vi "FeedBack Chanel.vi"(0 "Test Name":string, 5 "Channels (Int)":i32[](array[numeric]), 7 "FeedBack Channel":string[](array[string])=["fgdgfvcbc", "vnfhgjkn", "21354682"], 9 "Wait/Poll (ms)":u32, 11 "Parameter":u8) -> (4 "Out":i32, 6 "Array":bool[](array[boolean]), 8 "Fail":bool, 12 "Input Status":bool[](array[boolean]), 13 "Channel No":i32[](array[numeric]))   [LabVIEW 2015]
uses:
  Galobal variable_TI.vi
  Project Setup/Globle Variable/GR_Servo.vi
panel:
  in  "Load":bool
  out "Pokayoka Result":cluster{"Sensor Name":string, "Boolean":bool}[](array[cluster])
  out "output array":bool[](array[boolean])
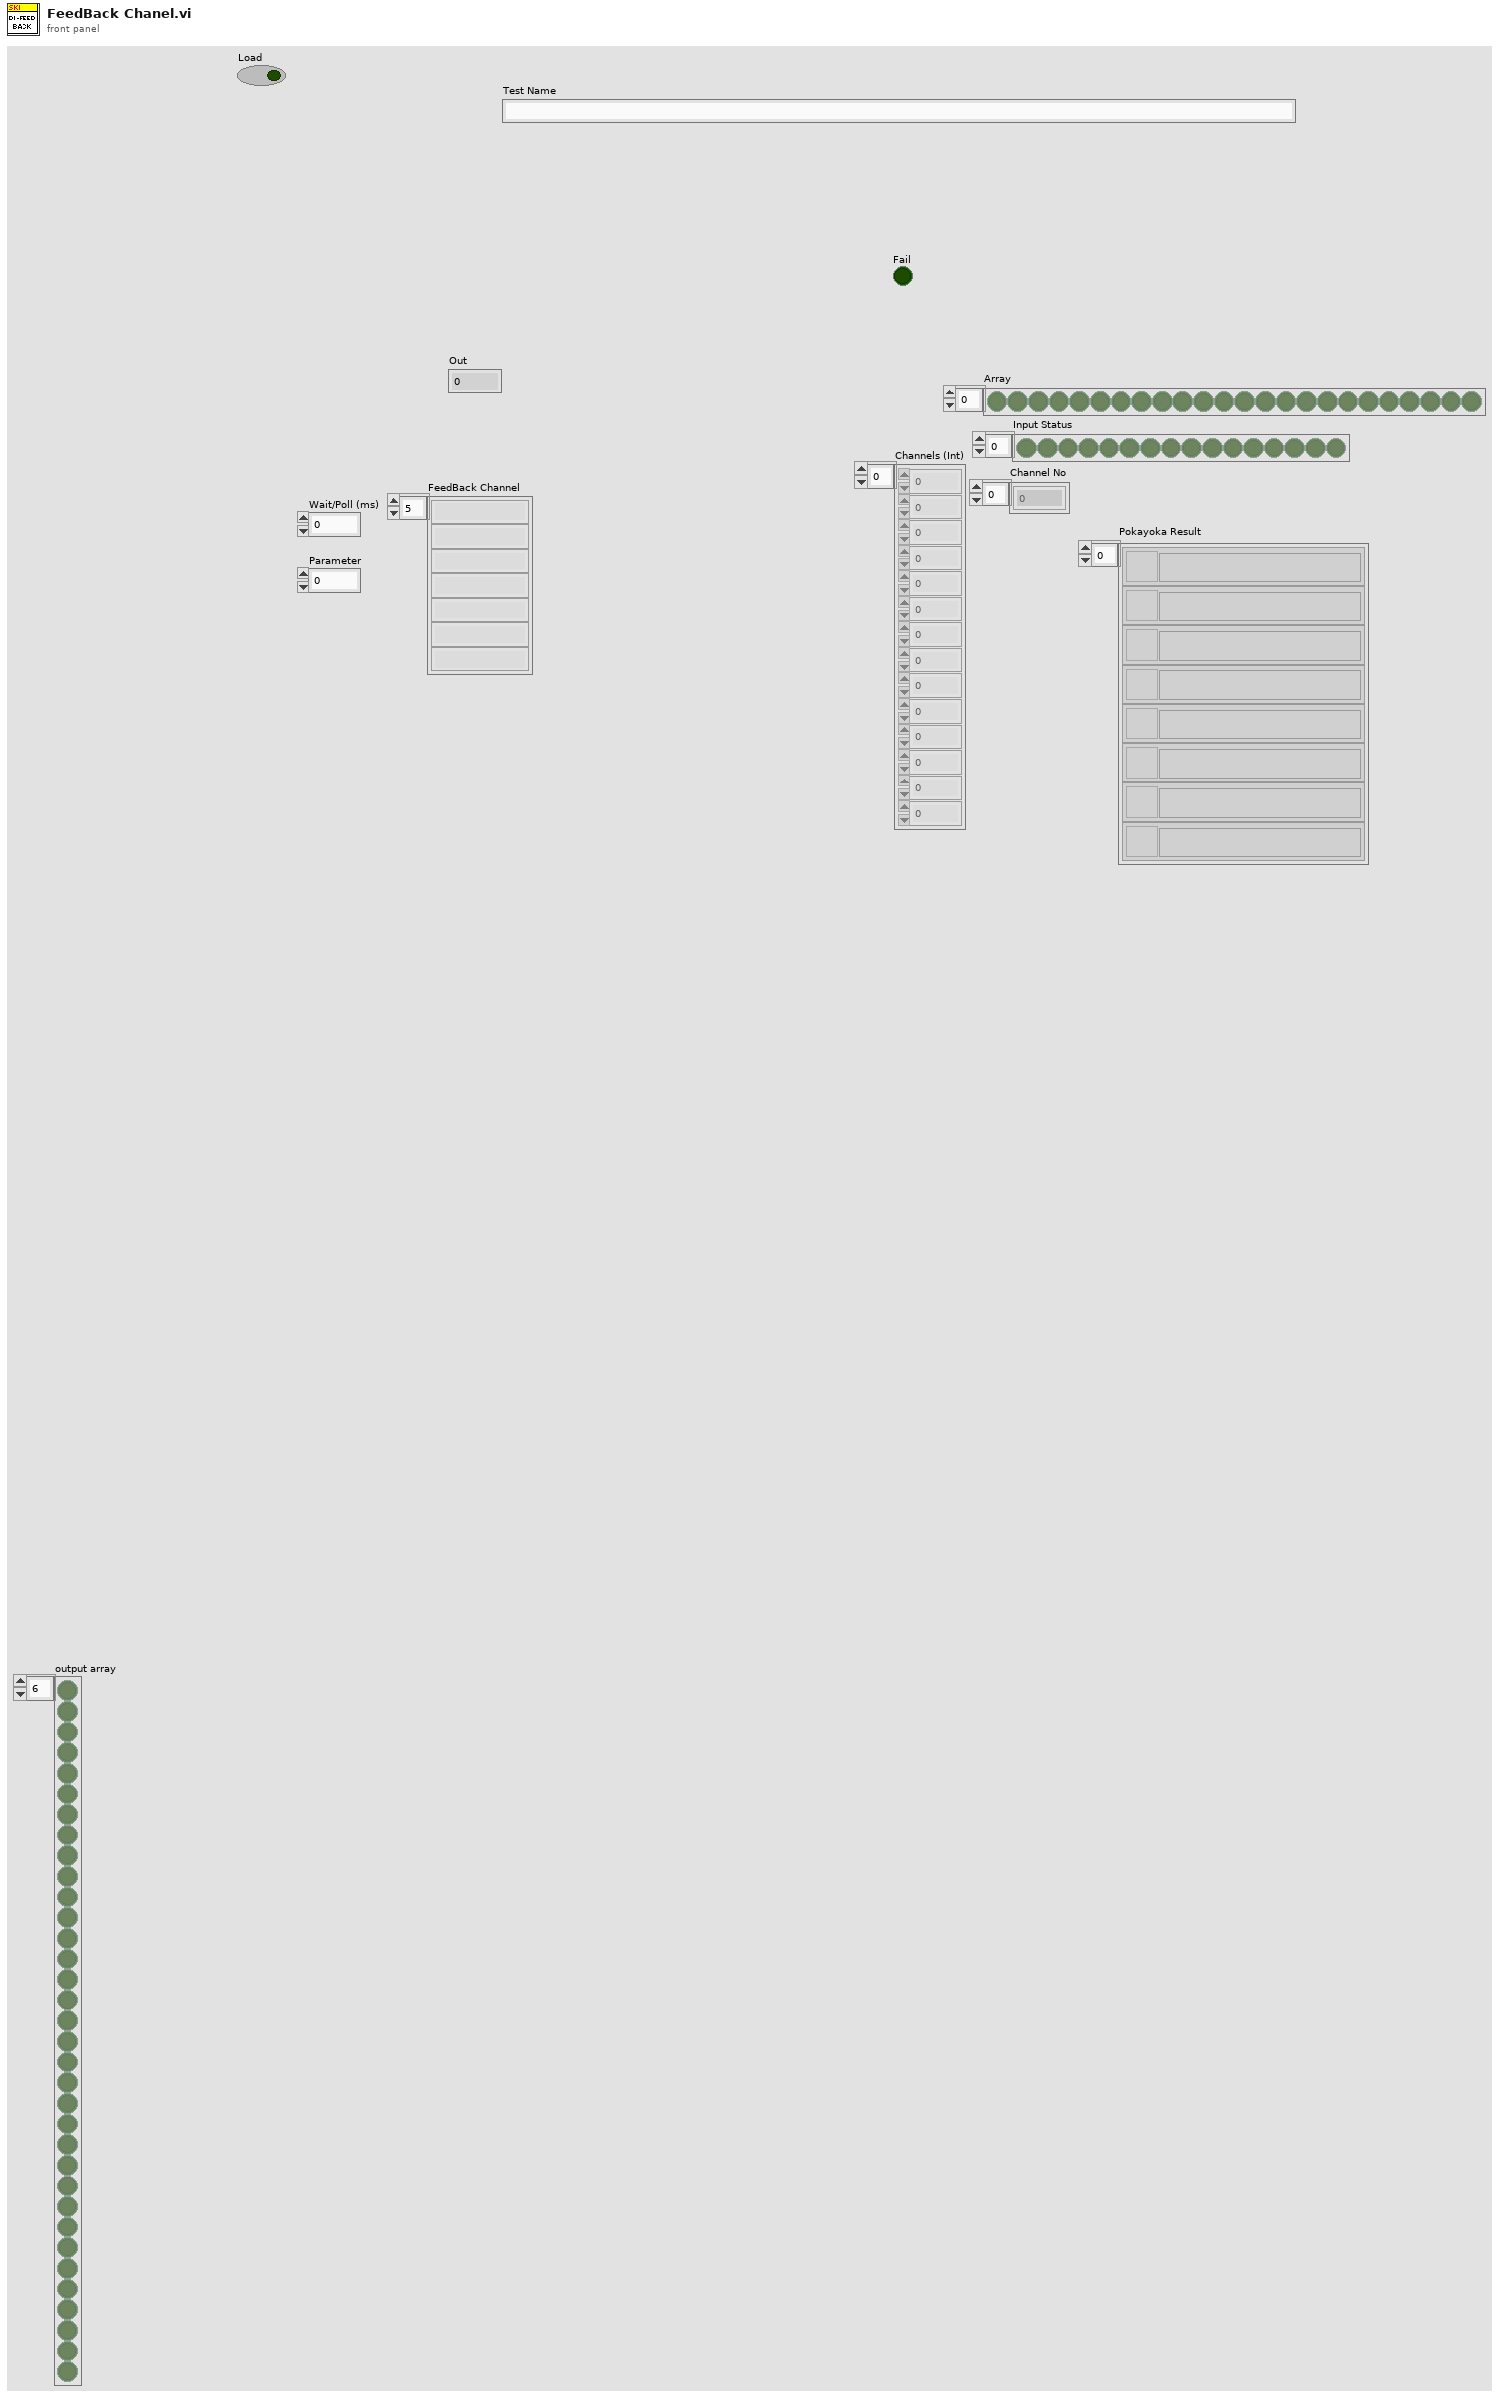
[diagram p1: front panel]
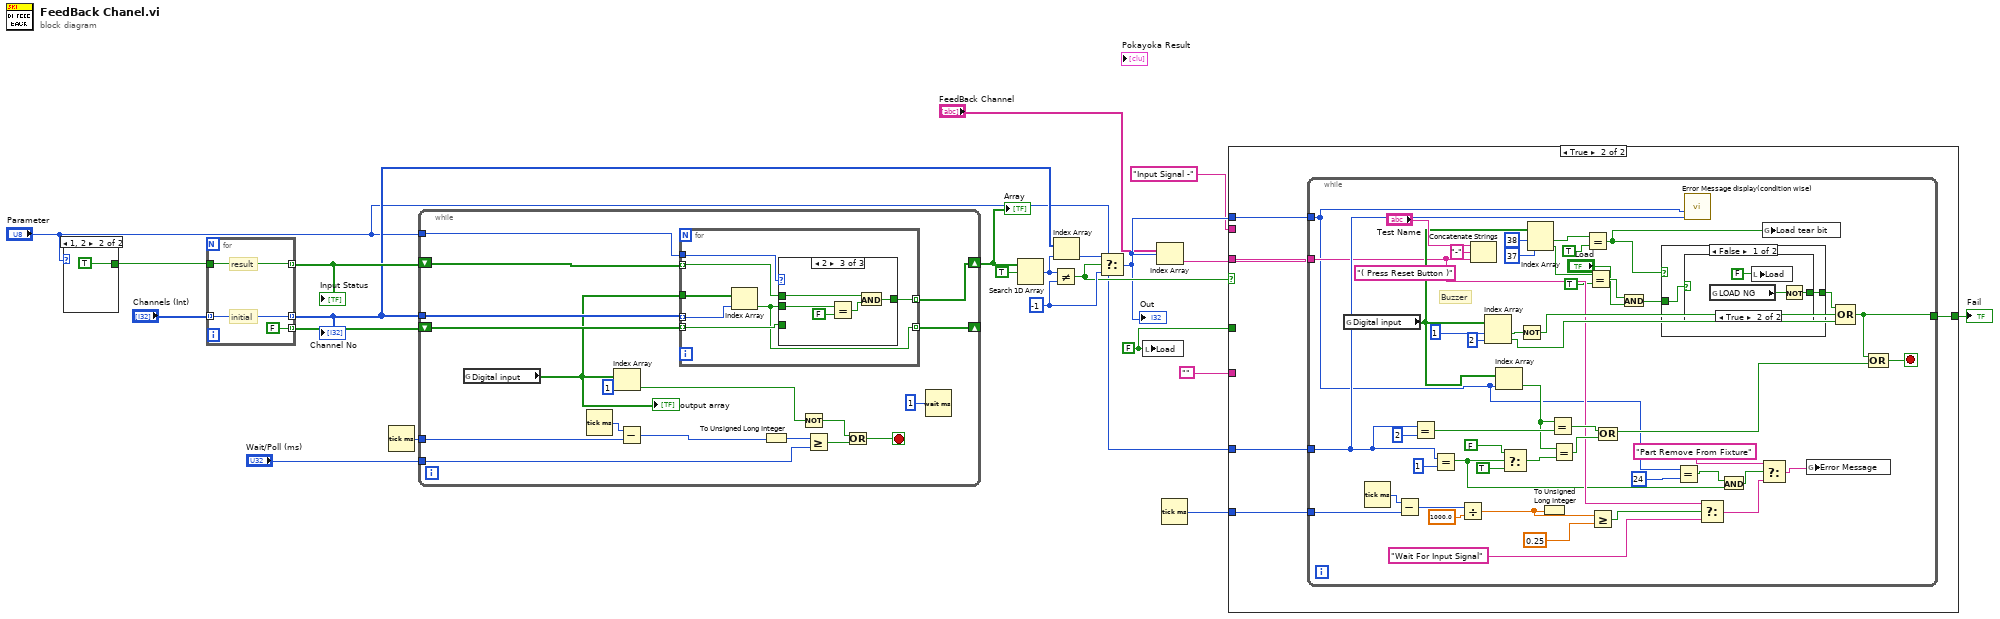
[diagram p0: block diagram]
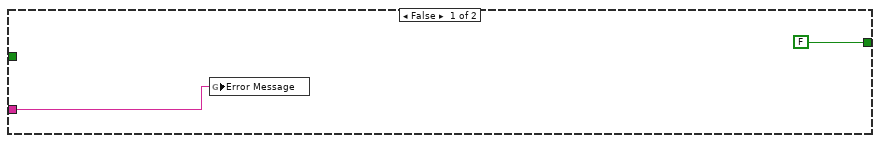
[diagram p2: hidden frame]
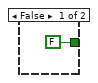
[diagram p3: hidden frame]
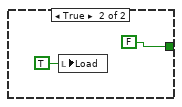
[diagram p4: hidden frame]
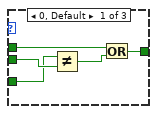
[diagram p5: hidden frame]
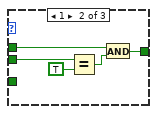
[diagram p6: hidden frame]
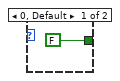
[diagram p7: hidden frame]
diagram:
  w1 = FALSE ("Load")
  w22 = -1 ("y")
  n1 = case shown="1, 2" "Parameter" {
    tunnel: [FALSE TRUE] -> w13
    frame 0, Default {
    }
    frame 1, 2 {
    }
  }
  n2 = for {
    tunnel: [w27] -> w8 mode=indexing
    tunnel: w13 -> [w27]
    tunnel: "Channels (Int)" -> [w26] mode=indexing
    tunnel: [w26] -> w7 mode=indexing
    tunnel: [FALSE] -> w17 mode=indexing
    # "result"
    # "initial"
  }
  "Input Status" <- w8
  "Channel No" <- w7
  n3 = Tick Count (ms)() -> (millisecond timer value=w16:u32)
  n4 = while {
    tunnel: "Wait/Poll (ms)" -> [w33]
    tunnel: w16 -> [w44]
    tunnel: w7 -> [w42]
    tunnel: "Parameter" -> [w41]
    shift-right: [w40] -> w19
    shift-left: w8 -> [w38]
    shift-right: [w39] -> _
    shift-left: w17 -> [w37]
    stop <- w35 stop-if-true
    n5 = global read "Galobal variable_TI.vi" "Digital input"() -> (w29:bool[])
    "output array" <- w29
    n6 = Tick Count (ms)() -> (millisecond timer value=w45:u32)
    n7 = Index Array(array=w29, index=1) -> (element=w31:bool)
    n8 = Subtract(x=w45, y=w44) -> (x-y=w28:u32)
    n9 = for {
      tunnel: w37 -> [w47] mode=indexing
      tunnel: w38 -> [w49] mode=indexing
      tunnel: w29 -> [w52]
      tunnel: w42 -> [w51] mode=indexing
      tunnel: w41 -> [w50]
      tunnel: [w48] -> w40 mode=indexing
      tunnel: [w46] -> w39 mode=indexing
      n10 = Index Array(array=w52, index=w51) -> (element=w46:bool)
      n11 = case shown="2" w50 {
        tunnel: w46 -> [w57 w60 w67]
        tunnel: w49 -> [w55 w59 w64]
        tunnel: [w53 w58 w63] -> w48
        tunnel: w47 -> [w56 _ _]
        frame 0, Default {
          n12 = Not Equal?(x=w56, y=w57) -> (x != y?=w54:bool)
          n13 = Or(x=w55, y=w54) -> (x .or. y?=w53:bool)
        }
        frame 1 {
          n14 = Equal?(x=w60, y=TRUE) -> (x = y?=w61:bool)
          n15 = And(x=w59, y=w61) -> (x .and. y?=w58:bool)
        }
        frame 2 {
          n16 = Equal?(x=w67, y=FALSE) -> (x = y?=w65:bool)
          n17 = And(x=w64, y=w65) -> (x .and. y?=w63:bool)
        }
      }
    }
    n18 = To Unsigned Long Integer(number=w28) -> (unsigned 32bit integer=w43:u32)
    n19 = Not(x=w31) -> (.not. x?=w32:bool)
    n20 = Greater Or Equal?(x=w43, y=w33) -> (x >= y?=w36:bool)
    n21 = Or(x=w32, y=w36) -> (x .or. y?=w35:bool)
    n22 = Wait (ms)(milliseconds to wait=u32 1) -> ()  [unwired: 1 out]
  }
  "Array" <- w19
  n23 = Search 1D Array(1D array=w19, element=TRUE) -> (index of element=w20:i32)  [unwired: 1 in]
  n24 = Not Equal?(x=w20, y=w22) -> (x != y?=w12:bool)
  n25 = Index Array(array=w7, index=w20) -> (element=w21:i32)
  n26 = Select(t=w21, s=w12, f=w22) -> (s? t:f=w11:i32)
  "Out" <- w11
  n27 = local write "Load"(w1) -> ()
  n28 = Index Array(array="FeedBack Channel", index=w11) -> (element=w10:string)
  n29 = Tick Count (ms)() -> (millisecond timer value=w5:u32)
  n30 = case shown="True" w12 {
    tunnel: w11 -> [_ w73]
    tunnel: w10 -> [_ w74]
    tunnel: "Input Signal -" ("string") -> [_ _]
    tunnel: w5 -> [_ w72]
    tunnel: "" -> [w69 _]
    tunnel: [FALSE w71] -> w2
    tunnel: "Parameter" -> [_ w70]
    tunnel: w1 -> [_ _]
    frame False {
      n31 = global write "GR_Servo.vi" "Error Message"(w69) -> ()
    }
    frame True {
      n32 = while {
        tunnel: w74 -> [w92]
        tunnel: w73 -> [w90]
        tunnel: w72 -> [w117]
        tunnel: [w98] -> w71
        tunnel: w70 -> [w97]
        stop <- w122 stop-if-true
        (unwired) "( Press Reset Button )" ("string")
        # "Buzzer"
        n33 = global read "Galobal variable_TI.vi" "Digital input"() -> (w96:bool[])
        n34 = Tick Count (ms)() -> (millisecond timer value=w120:u32)
        n35 = Subtract(x=w120, y=w117) -> (x-y=w119:u32)
        n36 = Equal?(x=w97, y=u8 2) -> (x = y?=w103:bool)
        n37 = Equal?(x=w97, y=u8 1) -> (x = y?=w88:bool)
        n38 = Divide(x=w119, y=1000.0) -> (x/y=w91:dbl)
        n39 = Concatenate Strings("Test Name", "-" ("string"), w92) -> ()  [unwired: 1 out]
        n40 = Index Array(array=w96, index #1=1 ("index"), index #2=2 ("index")) -> (element #1=w112:bool, element #2=w109:bool)
        n41 = Index Array(array=w96, index=w90) -> (element=w102:bool)
        n42 = Select(t=FALSE, s=w88, f=TRUE) -> (s? t:f=w104:bool)
        n43 = Not(x=w112) -> (.not. x?=w110:bool)
        n44 = Index Array(array=w96, index #1=38 ("index"), index #2=37 ("index")) -> (element #1=w94:bool, element #2=w79:bool)
        n45 = To Unsigned Long Integer(number=w91) -> ()  [unwired: 1 out]
        n46 = Equal?(x=w102, y=w103) -> (x = y?=w101:bool)
        n47 = Equal?(x=w102, y=w104) -> (x = y?=w100:bool)
        n48 = Equal?(x=w94, y=TRUE) -> (x = y?=w76:bool)
        n49 = Equal?(x=w79, y=TRUE) -> (x = y?=w78:bool)
        n50 = Greater Or Equal?(x=w91, y=0.25) -> (x >= y?=w115:bool)
        n51 = Compound Arithmetic op=OR(w101, w100) -> (w99:bool)
        n52 = And(x=w78, y="Load") -> (x .and. y?=w75:bool)
        n53 = case shown="False" w76 {
          tunnel: [w125 FALSE ("LOAD NG")] -> w82
          tunnel: w75 -> [w124 _]
          frame False {
            n54 = case shown="True" w124 {
              tunnel: [FALSE w128] -> w125
              frame False {
              }
              frame True {
                n55 = global read "Galobal variable_TI.vi" "LOAD NG"() -> (w129:bool)
                n56 = local write "Load"(FALSE ("Load")) -> ()
                n57 = Not(x=w129) -> (.not. x?=w128:bool)
              }
            }
          }
          frame True {
            n58 = local write "Load"(TRUE ("Load")) -> ()
          }
        }
        n59 = Equal?(x=w90, y=24) -> (x = y?=w87:bool)
        n60 = call "Error Message display(condition wise).vi"("Check Status(2-hi,1Lo,0 def"=w97, "Index No"=w90) -> ()  [unwired: 7 in, 1 out]
        n61 = Select(t=w92, s=w115, f="Wait For Input Signal") -> (s? t:f=w85:string)
        n62 = And(x=w87, y=w88) -> (x .and. y?=w86:bool)
        n63 = Select(t="Part Remove From Fixture", s=w86, f=w85) -> (s? t:f=w83:string)
        n64 = global write "Galobal variable_TI.vi" "Load tear bit"(w76) -> ()
        n65 = global write "GR_Servo.vi" "Error Message"(w83) -> ()
        n66 = Compound Arithmetic op=OR(w82, w110, w109) -> (w98:bool)
        n67 = Compound Arithmetic op=OR(w98, w99) -> (w122:bool)
      }
    }
  }
  "Fail" <- w2
